vi "TWO_BOTTON_TO_ONE(SubVI).vi"(1 "Boton 2":refnum<vi>, 2 "Boton 2":u16, 3 "Boton 1":u16, 4 "Boton 1":refnum<vi>) -> (0 "Value":u16)   [LabVIEW 2011]
doc: "Escribe el valor del boton que cambia sobre el que no cambia, y saca el valor. Para comprender mejor mirar bloque de diagrama."
uses:
  U16 Changed__ogtk.vi
panel:
  # "Escribe el valor del boton que cambia sobre el que no cambia, y saca el valor."
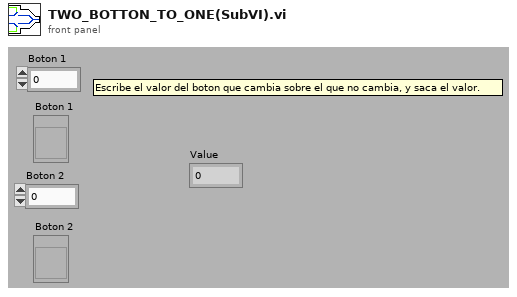
[diagram p1: front panel]
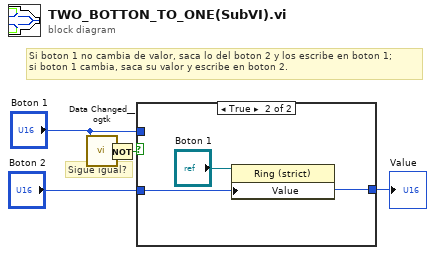
[diagram p0: block diagram]
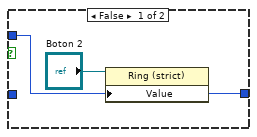
[diagram p2: hidden frame]
diagram:
  # "Sigue igual?"
  # "Si boton 1 no cambia de valor, saca lo del boton 2 y los escribe en boton 1;\nsi boton 1 cambia, saca su valor y escribe en boton 2."
  n1 = call-poly "Data Changed__ogtk.vi"("U16"="Boton 1") -> ("Changed"=w1:bool)
  n2 = Not(x=w1) -> (.not. x?=w5:bool)
  n3 = case shown="True" w5 {
    tunnel: [w6 w9] -> w2
    tunnel: "Boton 1" -> [w6 _]
    tunnel: "Boton 2" -> [_ w9]
    frame False {
      n4 = property on="Property Node" class="Ring (strict)"(reference="Boton 2", "Value"=w6) -> ()  [unwired: 1 in, 2 out]
    }
    frame True {
      n5 = property on="Property Node" class="Ring (strict)"(reference="Boton 1", "Value"=w9) -> ()  [unwired: 1 in, 2 out]
    }
  }
  "Value" <- w2
